vi "Setup.vi"(0 "SA Path Group in":refnum<class "SA Path Group.lvclass">, 11 "error in":errorcluster) -> (4 "SA Path Group out":refnum<class "SA Path Group.lvclass">, 15 "error out":errorcluster)   [LabVIEW 2023, in "RFFixtureCharact.PXI.lvlib" / "SA Path Group.lvclass"]
uses:
  SA Path Group.lvclass
  SA Path Group.lvclass/SA Path Group.ctl
  Public/Base Classes/Scalar/Scalar Path/Scalar Path.lvclass
  Common/RFCalAndFixtureCharact.Common.lvlib
  Public/Base Classes/Scalar/Scalar Path Group/Scalar Path Group.lvclass
  Public/Base Classes/Scalar/SA Path/SA Path.lvclass
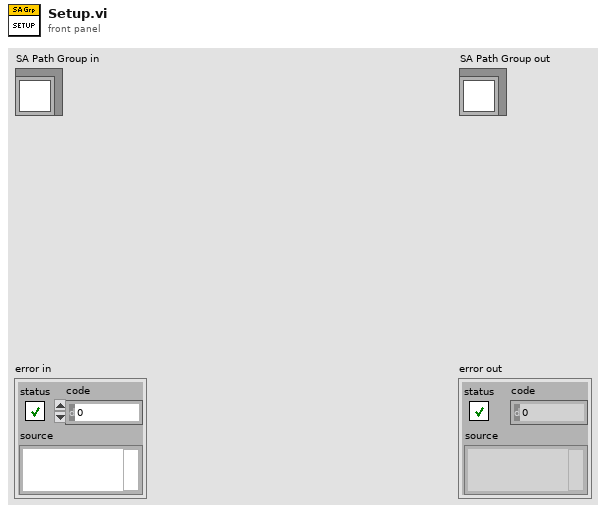
[diagram p1: front panel]
types:
  T1 = typedef "RFFixtureCharact.Public.lvlib/Scalar Path Group.lvclass/Sweep.ctl" = cluster{"Port Power":dbl, "Frequencies":dbl[], "Reference Level":dbl}
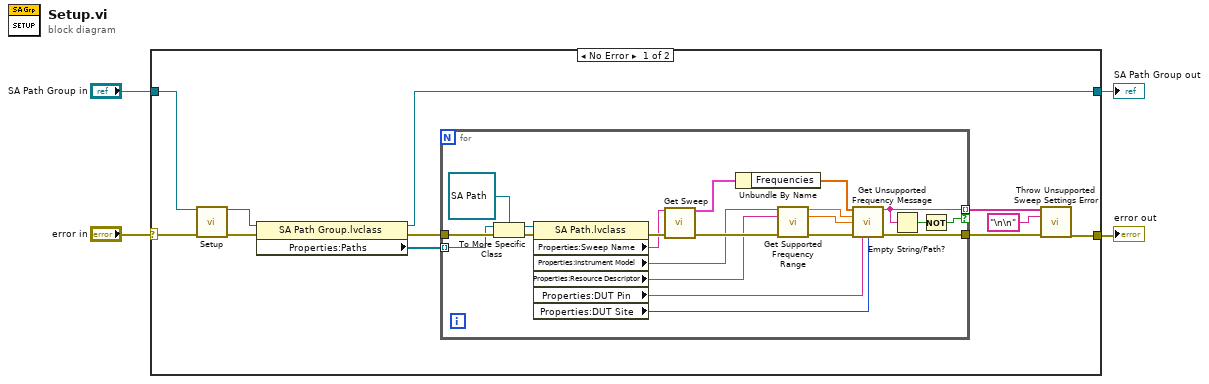
[diagram p0: block diagram]
diagram:
  n1 = case shown="No Error" "error in" {
    selector: "error in" -> [w9 w38]
    tunnel: "SA Path Group in" -> [w15 w37]
    tunnel: [w7 w38] -> w3
    tunnel: [w10 w37] -> w2
    frame No Error {
      n2 = call-parent "Setup.vi"("Path Group in"=w15, "error in"=w9) -> ("Path Group out"=w11:refnum<class "SA Path Group.lvclass">, "error out"=w12:errorcluster)  [unwired: 12 in]
      n3 = property class="SA Path Group.lvclass"(reference=w11, error in=w12) -> (reference out=w10:refnum<class "SA Path Group.lvclass">, error out=w13:errorcluster, "Properties:Paths"=w14:refnum<class "Path.lvclass">[])
      n4 = for {
        tunnel: w14 -> [w35] mode=indexing
        tunnel: w13 -> [w36]
        tunnel: [w24] -> w8
        tunnel: [w16] -> w5 mode=indexing if=w17
        n5 = To More Specific Class(target class=refnum<class "SA Path.lvclass"> refnum ("RFFixtureCharact.Public.lvlib:SA Path.lvclass"), reference=w35, error in=w36) -> (specific class reference=w34:refnum<class "SA Path.lvclass">, error out=w33:errorcluster)
        n6 = property class="SA Path.lvclass"(reference=w34, error in=w33) -> (error out=w32:errorcluster, "Properties:Sweep Name"=w31:string, "Properties:Instrument Model"=w27:string, "Properties:Resource Descriptor"=w26:string, "Properties:DUT Pin"=w21:string, "Properties:DUT Site"=w20:i32)  [unwired: 1 out]
        n7 = call "Get Sweep.vi"("Sweep Name"=w31, "error in (no error)"=w32) -> ("Sweep"=w30:T1, "error out"=w28:errorcluster)  [unwired: 11 in, 1 out]
        n8 = Unbundle By Name(w30) -> ("Frequencies"=w19:dbl[])
        n9 = call "Get Supported Frequency Range.vi"("Instrument Model"=w27, "Instrument Name"=w26, "error in"=w28) -> ("Maximum Frequency"=w23:dbl, "Minmum Frequency"=w22:dbl, "error out"=w25:errorcluster)  [unwired: 10 in]
        n10 = call "Get Unsupported Frequency Message.vi"("Frequencies"=w19, "Maximum Frequency"=w23, "Minimum Frequency"=w22, "error in"=w25, "DUT Pin"=w21, "DUT Site"=w20) -> ("Unspported Frequency Message"=w16:string, "error out"=w24:errorcluster)  [unwired: 8 in]
        n11 = Empty String/Path?(string/path=w16) -> (empty?=w18:bool)
        n12 = Not(x=w18) -> (.not. x?=w17:bool)
      }
      n13 = call "Throw Unsupported Sweep Settings Error.vi"("Error Message List"=w5, "Delimiter ('\\n')"="\n\n" ("Paths Error Message Delimiter"), "error in"=w8) -> ("error out"=w7:errorcluster)  [unwired: 12 in]
    }
    frame Error {
    }
  }
  "error out" <- w3
  "SA Path Group out" <- w2
